vi "未命名 7.vi"() -> ()   [LabVIEW 2016]
uses:
  Beverage/CondimentDecorator/Mocha/Mocha.lvclass
  Beverage/CondimentDecorator/Soy/Soy.lvclass
  Beverage/House Blend Coffee/House Blend Coffee.lvclass
  Beverage/Espresso/Espresso.lvclass
  Beverage/Beverage.lvclass
panel:
  in  "加入Soy":bool
  in  "加入Mocha":bool
  in  "枚举":enum16{"1", "2"}(ring)=enum."2"
  out "连接的字符串":string
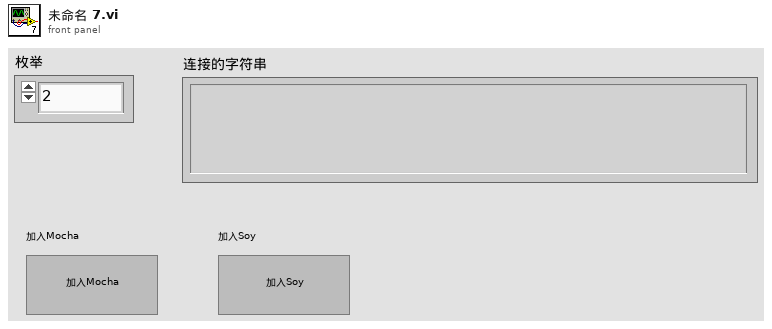
[diagram p1: front panel]
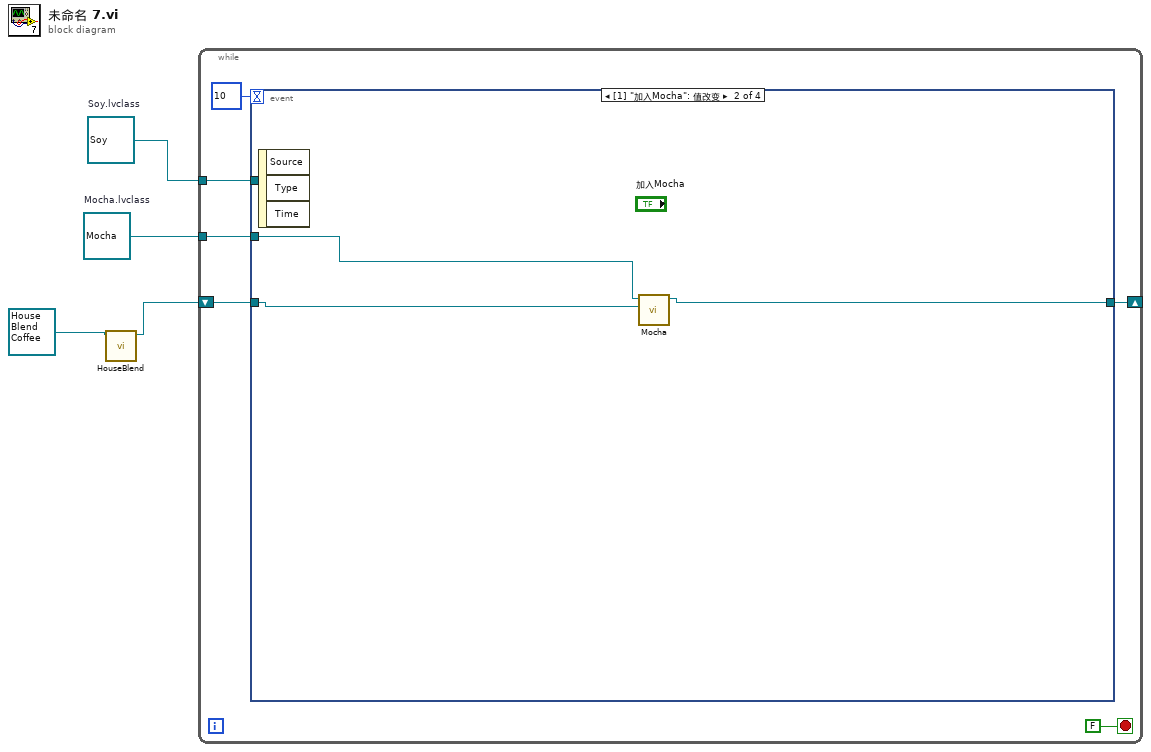
[diagram p0: block diagram]
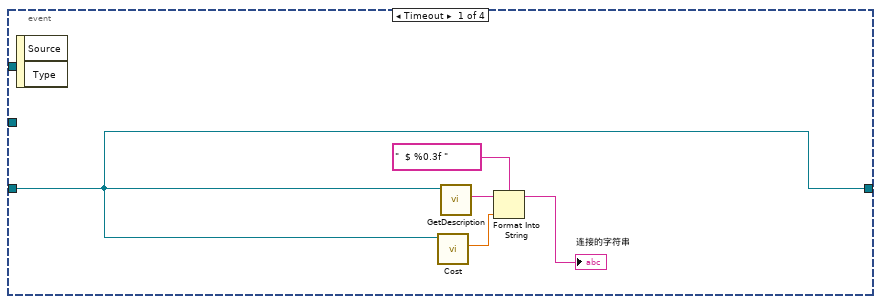
[diagram p2: hidden frame]
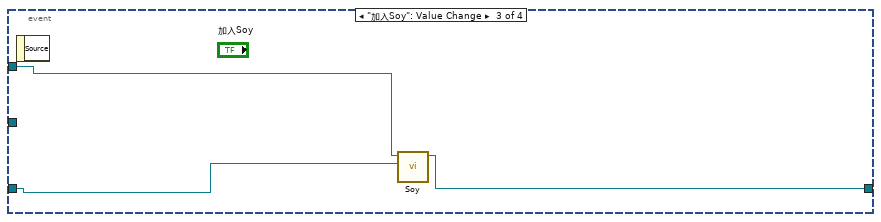
[diagram p3: hidden frame]
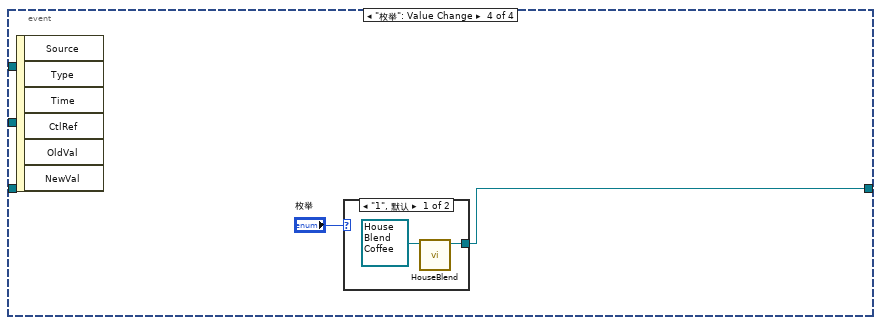
[diagram p4: hidden frame]
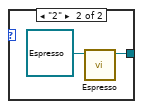
[diagram p5: hidden frame]
diagram:
  w3 = refnum<class "Soy.lvclass"> refnum  # Soy.lvclass
  w4 = refnum<class "Mocha.lvclass"> refnum  # Mocha.lvclass
  n1 = call "HouseBlend.vi"("House Blend Coffee 输入"=refnum<class "House Blend Coffee.lvclass"> refnum ("House Blend Coffee.lvclass")) -> ("House Blend Coffee 输出"=w1:refnum<class "House Blend Coffee.lvclass">)  [unwired: 9 in, 1 out]
  n2 = while {
    shift-right: [w8] -> _
    shift-left: w1 -> [w7]
    tunnel: w4 -> [w6]
    tunnel: w3 -> [w5]
    stop <- FALSE stop-if-true
    n3 = event shown="[1] \"加入Mocha\": 值改变" {
      selector: _ -> [_ _ _ _]
      dyn-events: _ -> [_ _ _ _]
      timeout: 10 -> [_ _ _ _]
      tunnel: [w11 w17 w20 w22] -> w8
      tunnel: w7 -> [w11 w18 w21 _]
      tunnel: w6 -> [_ w16 _ _]
      tunnel: w5 -> [_ _ w19 _]
      event Timeout {
        n4 = event-data() -> ()  [unwired: 1 in, 2 out]
        n5 = call-dynamic "Cost.vi"("Beverage 输入"=w11) -> ("cost"=w14:dbl)  [unwired: 8 in, 2 out]
        n6 = call-dynamic "GetDescription.vi"("Beverage 输入"=w11) -> ("Description"=w12:string)  [unwired: 8 in, 2 out]
        n7 = Format Into String(format string="  $ %0.3f " ("字符串"), initial string=w12, w14) -> (resulting string=→"连接的字符串":string)  [unwired: 1 in, 1 out]
      }
      event "加入Mocha": Value Change {
        n8 = event-data() -> ()  [unwired: 1 in, 3 out]
        n9 = call "Mocha.vi"("Beverage.lvclass"=w18, "Mocha 输入"=w16) -> ("Mocha 输入"=w17:refnum<class "Mocha.lvclass">)  [unwired: 8 in, 1 out]
      }
      event "加入Soy": Value Change {
        n10 = event-data() -> ()  [unwired: 1 in, 1 out]
        n11 = call "Soy.vi"("Beverage.lvclass"=w21, "Soy 输入"=w19) -> ("Soy 输入"=w20:refnum<class "Soy.lvclass">)  [unwired: 8 in, 1 out]
      }
      event "枚举": Value Change {
        n12 = event-data() -> ()  [unwired: 1 in, 6 out]
        n13 = case shown="\"1\", 默认" "枚举" {
          tunnel: [w24 w26] -> w22
          frame "1", Default {
            n14 = call "HouseBlend.vi"("House Blend Coffee 输入"=refnum<class "House Blend Coffee.lvclass"> refnum ("House Blend Coffee.lvclass")) -> ("House Blend Coffee 输出"=w24:refnum<class "House Blend Coffee.lvclass">)  [unwired: 9 in, 1 out]
          }
          frame "2" {
            n15 = call "Espresso.vi"("Espresso 输入"=refnum<class "Espresso.lvclass"> refnum ("Espresso.lvclass")) -> ("Espresso 输出"=w26:refnum<class "Espresso.lvclass">)  [unwired: 9 in, 1 out]
          }
        }
      }
    }
  }
